vi "UpdateSnakeOnBoard.vi"(0 "object in":refnum<class "Game Board.lvclass">, 5 "error in (no error)":errorcluster) -> (14 "object out":refnum<class "Game Board.lvclass">, 19 "error out":errorcluster)   [LabVIEW 2021, in "Game Board.lvclass"]
uses:
  Game Board.lvclass
  Game Board.lvclass/Game Board.ctl
  Snake_class/Snake.lvclass
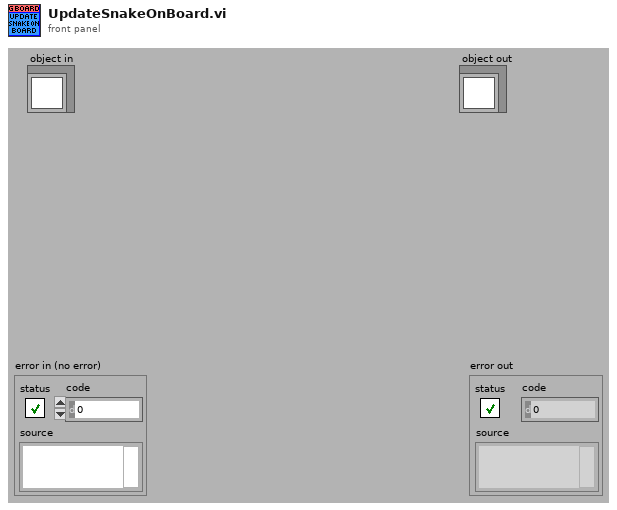
[diagram p1: front panel]
types:
  T1 = typedef "Coordinates.ctl" = cluster{"X":i32, "Y":i32}
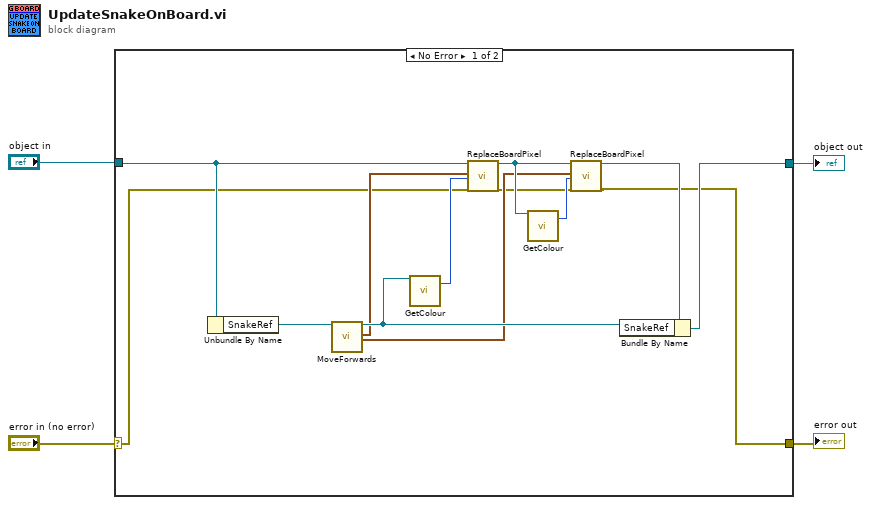
[diagram p0: block diagram]
diagram:
  n1 = case shown="No Error" "error in (no error)" {
    selector: "error in (no error)" -> [w7 w19]
    tunnel: [w5 w19] -> w3
    tunnel: [w17 w18] -> w1
    tunnel: "object in" -> [w14 w18]
    frame No Error {
      n2 = Unbundle By Name(w14) -> ("SnakeRef"=w16:refnum<class "Snake.lvclass">)
      n3 = call-dynamic "MoveForwards.vi"("object in"=w16) -> ("object out"=w15:refnum<class "Snake.lvclass">, "New Head"=w12:T1, "Deleted Tail"=w8:T1)  [unwired: 15 in, 1 out]
      n4 = call-dynamic "GetColour.vi"("object in"=w15) -> ("Colour"=w13:u32)  [unwired: 16 in, 2 out]
      n5 = call-dynamic "ReplaceBoardPixel.vi"("object in"=w14, "Coordinates"=w12, "Colour"=w13, "error in (no error)"=w7) -> ("object out"=w10:refnum<class "Game Board.lvclass">, "error out"=w6:errorcluster)  [unwired: 14 in]
      n6 = call-dynamic "GetColour.vi"("object in"=w10) -> ("Colour"=w9:u32)  [unwired: 16 in, 2 out]
      n7 = call-dynamic "ReplaceBoardPixel.vi"("object in"=w10, "Coordinates"=w8, "Colour"=w9, "error in (no error)"=w6) -> ("object out"=w11:refnum<class "Game Board.lvclass">, "error out"=w5:errorcluster)  [unwired: 14 in]
      n8 = Bundle By Name(cluster=w11, "SnakeRef"=w15) -> (w17:refnum<class "Game Board.lvclass">)
    }
    frame Error {
    }
  }
  "error out" <- w3
  "object out" <- w1
